vi "Temperature Warnings.vi"(8 "Error In":errorcluster, 9 "Min Temperature":dbl, 10 "Max Temperature":dbl, 11 "Current Temperature":dbl) -> (0 "Error Out":errorcluster, 2 "Warning Text":string="No Warning", 3 "Warning?":bool)   [LabVIEW 2015]
doc: "This VI is used to determine the string to output to the weather station based on the current temperature and limit settings.\n\nInputs: Current Temperature (DBL), Minimum Temperature (DBL), and Maximum Temperature (DBL).\nOutputs: Warning Text (string) and Warning? (Boolean)."
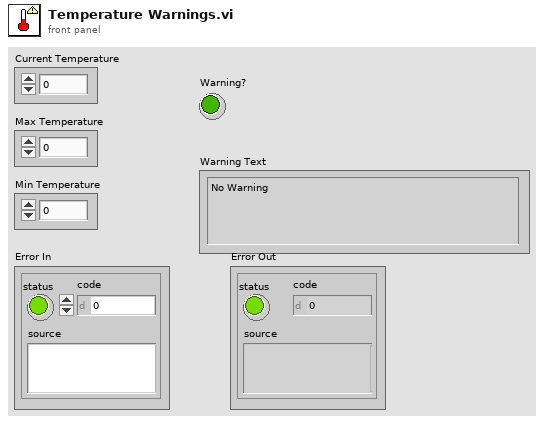
[diagram p1: front panel]
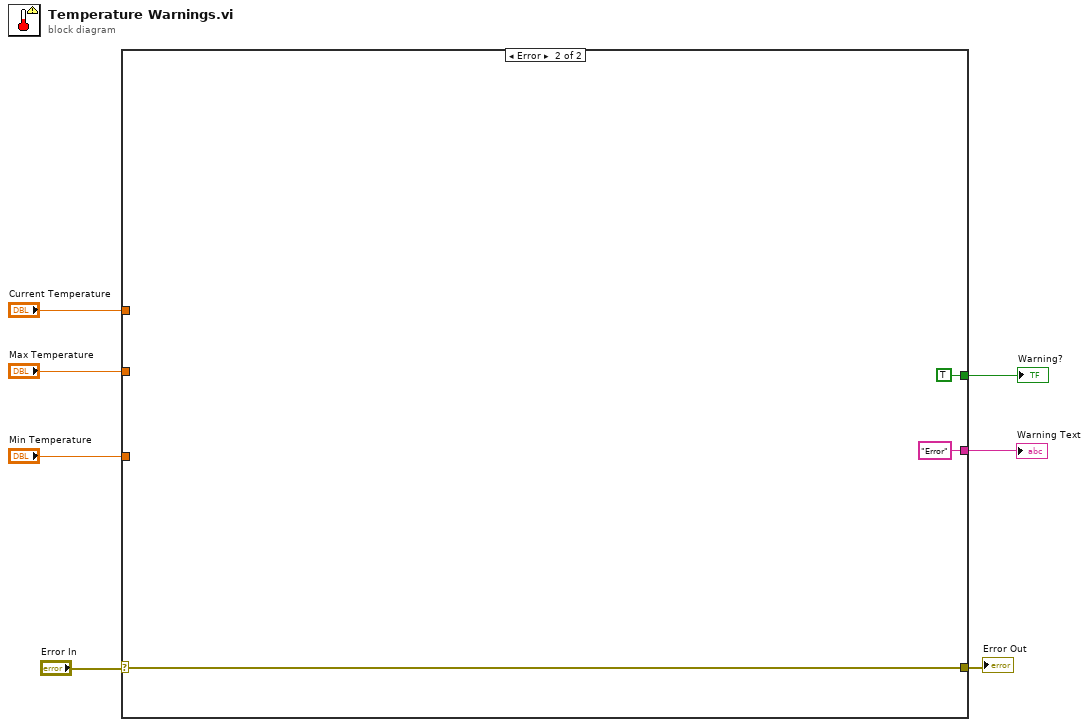
[diagram p0: block diagram]
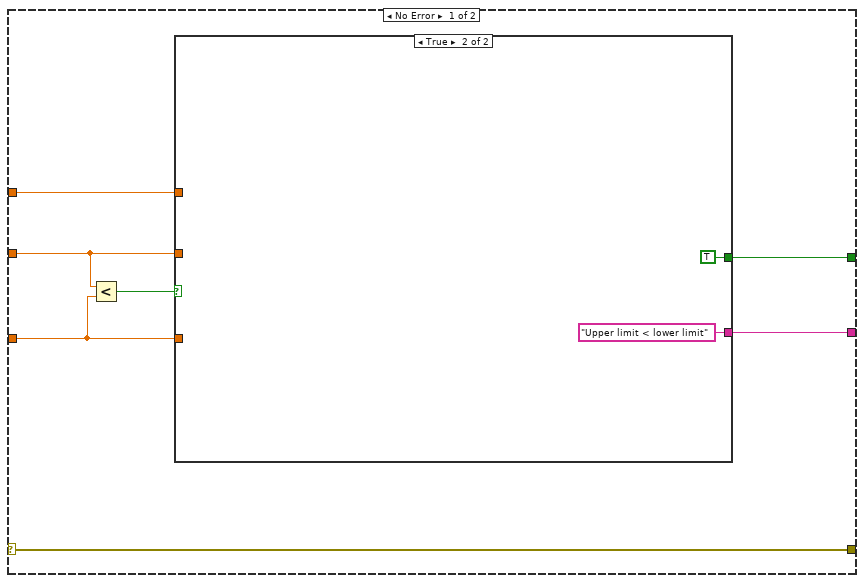
[diagram p2: hidden frame]
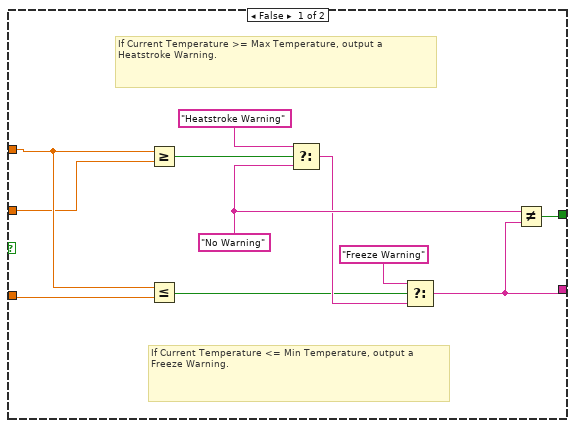
[diagram p3: hidden frame]
diagram:
  n1 = case shown="Error" "Error In" {
    selector: "Error In" -> [w11 w30]
    tunnel: "Current Temperature" -> [w14 _]
    tunnel: "Min Temperature" -> [w9 _]
    tunnel: "Max Temperature" -> [w10 _]
    tunnel: [w13 TRUE] -> w4
    tunnel: [w12 "Error" ("f")] -> w3
    tunnel: [w11 w30] -> w1
    frame No Error {
      n2 = Less?(x=w10, y=w9) -> (x < y?=w8:bool)
      n3 = case shown="True" w8 {
        tunnel: w14 -> [w19 _]
        tunnel: [w16 TRUE] -> w13
        tunnel: [w15 "Upper limit < lower limit" ("f")] -> w12
        tunnel: w10 -> [w17 _]
        tunnel: w9 -> [w18 _]
        frame False {
          w25 = "No Warning" ("f")
          # "If Current Temperature >= Max Temperature, output a Heatstroke Warning."
          # "If Current Temperature <= Min Temperature, output a Freeze Warning."
          n4 = Greater Or Equal?(x=w19, y=w17) -> (x >= y?=w20:bool)
          n5 = Less Or Equal?(x=w19, y=w18) -> (x <= y?=w23:bool)
          n6 = Select(t="Heatstroke Warning", s=w20, f=w25) -> (s? t:f=w24:string)
          n7 = Select(t="Freeze Warning", s=w23, f=w24) -> (s? t:f=w15:string)
          n8 = Not Equal?(x=w25, y=w15) -> (x != y?=w16:bool)
        }
        frame True {
        }
      }
    }
    frame Error {
    }
  }
  "Warning?" <- w4
  "Warning Text" <- w3
  "Error Out" <- w1
